vi "Select Custom Device.vi"(10 "CD Path":string, 11 "NIVS.System Definition Root":refnum<k24>) -> (1 "Cancelled?":bool, 2 "IP Address":string="Targets/Controller/Custom Devices/Communication Example", 3 "Custom Device Path Out":string="Targets/Controller/Custom Devices/Communication Example")   [LabVIEW 2023, in "J1939 Workspace Shared.lvlib"]
uses:
  J1939 Workspace Shared.lvlib
  NationalInstruments.VeriStand.SystemStorage
panel:
  in  "Cancel":bool
  in  "Select":bool
  in  "Custom Device Path":string(tree)
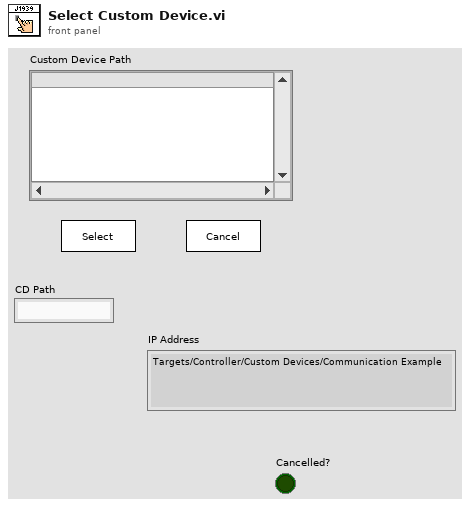
[diagram p1: front panel]
types:
  T1 = enum8{"Enabled", "Disabled", "Disabled and Grayed Out"}
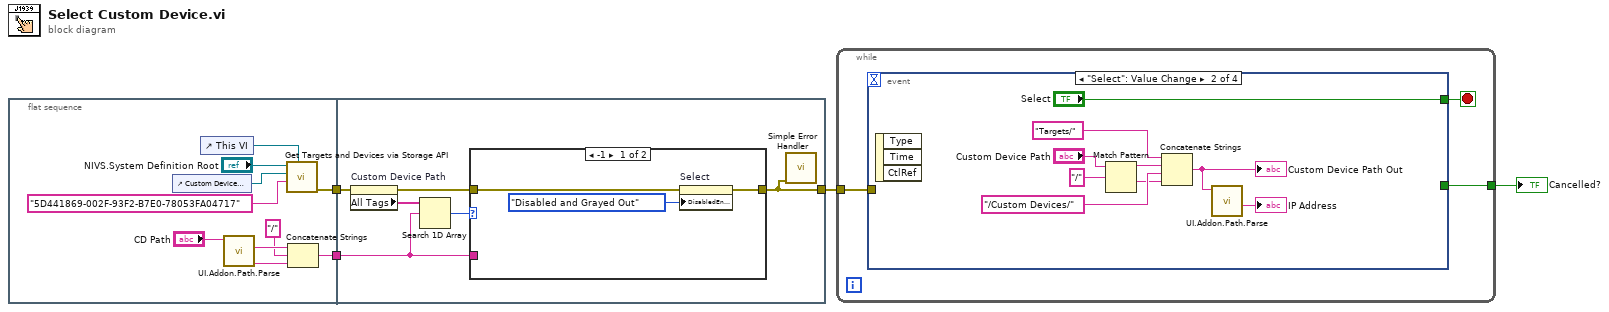
[diagram p0: block diagram]
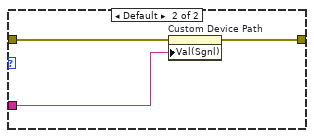
[diagram p2: hidden frame]
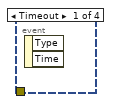
[diagram p3: hidden frame]
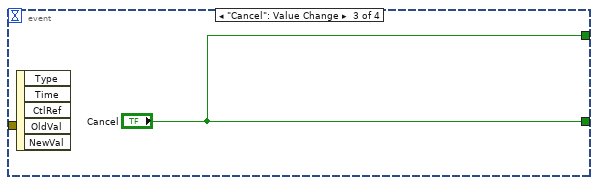
[diagram p4: hidden frame]
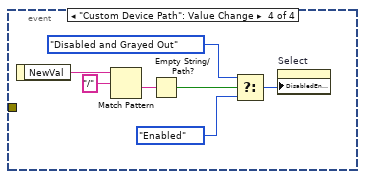
[diagram p5: hidden frame]
diagram:
  n1 = flat-sequence {
    tunnel: [w11] -> w3
    tunnel: [w9] -> w1
    tunnel: [w20] -> w4
    tunnel: w3 -> [w19]
    tunnel: w1 -> [w16]
    frame #0 {
      n2 = control-ref of="Custom Device Path"() -> (w13:refnum<vi>)
      n3 = control-ref of="This VI"() -> (w10:refnum<vi>)
      n4 = call "UI.Addon.Path.Parse.vi"("Cached Addon Path"="CD Path") -> ("Addon Name"=w6:string, "Controller and IP Address"=w7:string)  [unwired: 6 in, 3 out]
      n5 = call "Get Targets and Devices via Storage API.vi"("VI reference (current VI)"=w10, "Main GUID"="5D441869-002F-93F2-B7E0-78053FA04717", "Tree"=w13, "NIVS.System Definition Root"="NIVS.System Definition Root") -> ("error out"=w11:errorcluster)  [unwired: 6 in, 1 out]
      n6 = Concatenate Strings(w7, "/" ("string"), w6) -> (w9:string)
    }
    frame #1 {
      n7 = property on="Custom Device Path" class="Tree (strict)"(error in=w19) -> (error out=w18:errorcluster, "All Tags"=w17:string[])  [unwired: 1 in, 1 out]
      n8 = Search 1D Array(1D array=w17, element=w16) -> (index of element=w15:i32)  [unwired: 1 in]
      n9 = case shown="-1" w15 {
        tunnel: [w23 w26] -> w20
        tunnel: w18 -> [w22 w25]
        tunnel: w16 -> [_ w24]
        frame -1 {
          n10 = property on="Select" class="Bool"(error in=w22, "DisabledEnum"=T1."Disabled and Grayed Out" ("Disabled")) -> (error out=w23:errorcluster)  [unwired: 1 in, 1 out]
        }
        frame Default {
          n11 = property on="Custom Device Path" class="Tree (strict)"(error in=w25, "Val(Sgnl)"=w24) -> (error out=w26:errorcluster)  [unwired: 1 in, 1 out]
        }
      }
      n12 = call <vilib>:"Simple Error Handler.vi"("error in (no error)"=w20) -> ()  [unwired: 4 in, 5 out]
    }
  }
  n13 = while {
    tunnel: w4 -> [w29]
    tunnel: [w27] -> w2
    stop <- w28 stop-if-true
    n14 = event shown="[1] \"Select\": Value Change" {
      selector: _ -> [_ _ _ _]
      dyn-events: _ -> [_ _ _ _]
      timeout: _ -> [_ _ _ _]
      tunnel: w29 -> [_ _ _ _]
      tunnel: [_ "Select" "Cancel" _] -> w28
      tunnel: [_ _ "Cancel" _] -> w27
      event Timeout {
        n15 = event-data() -> ()  [unwired: 1 in, 2 out]
      }
      event "Select": Value Change {
        n16 = event-data() -> ()  [unwired: 1 in, 3 out]
        n17 = Match Pattern(string="Custom Device Path", regular expression="/") -> (before substring=w36:string, after substring=w34:string)  [unwired: 1 in, 2 out]
        n18 = Concatenate Strings("Targets/" ("string"), w36, "/Custom Devices/" ("string"), w34) -> (w31:string)
        "Custom Device Path Out" <- w31
        n19 = call "UI.Addon.Path.Parse.vi"("Cached Addon Path"=w31) -> ("IP Address"=→"IP Address":string)  [unwired: 6 in, 4 out]
      }
      event "Cancel": Value Change {
        n20 = event-data() -> ()  [unwired: 1 in, 5 out]
      }
      event "Custom Device Path": Value Change {
        n21 = event-data() -> ("NewVal"=w45:string)  [unwired: 1 in]
        n22 = Match Pattern(string=w45, regular expression="/") -> (after substring=w44:string)  [unwired: 1 in, 3 out]
        n23 = Empty String/Path?(string/path=w44) -> (empty?=w43:bool)
        n24 = Select(t=T1."Disabled and Grayed Out" ("Disabled"), s=w43, f=T1."Enabled" ("Disabled")) -> (s? t:f=w40:T1)
        n25 = property on="Select" class="Bool"("DisabledEnum"=w40) -> ()  [unwired: 2 in, 2 out]
      }
    }
  }
  "Cancelled?" <- w2
